vi "Configuration.Writer.Test.vi"() -> ()   [LabVIEW 2017, in "Measurement.Free.lvclass"]
uses:
  Measurement.Free.lvclass
  Typedefs/Configuration--Cluster.ctl
  Typedefs/Configuration.Hardware--Cluster.ctl
  Typedefs/Configuration.SMU--Cluster.ctl
  SMU/Typedefs/Configuration--Cluster.ctl
  Typedefs/Configuration.LIA--Cluster.ctl
  LIA/Typedefs/Configuration--Cluster.ctl
  Typedefs/Configuration.OPM--Cluster.ctl
  OPM/Typedefs/Configuration--Cluster.ctl
  Typedefs/Configuration.OPA--Cluster.ctl
  OPA/Typedefs/Configuration--Cluster.ctl
  <vilib>/Utility/config.llb/NI_LVConfig.lvlib
  SMU/SMU.lvclass
  LIA/LIA.lvclass
  OPM/OPM.lvclass
  OPA/OPA.lvclass
panel:
  out "error out":errorcluster
  in  "Configuration":T1={"Measurement.Type"=enum."Free", "Configuration.Hardware"={"Configuration.SMU"={"SMU Model"="Keithley2600", "Configuration"={"VISA Resource"="GPIB0::26::INSTR", "Channel"="A"}}, "Configuration.LIA"={"LIA Model"="SR810", "Configuration"={"VISA Resource"="GPIB0::8::INSTR"}}, "Configuration.OPM"={"OPM Model"="ThorlabsPM400", "Configuration"={"VISA Resource"="USB0::0x1313::0x8075::P5001221::INSTR"}}, "Configuration.OPA"={"OPA Model"="OrpheusHP", "Configuration"={"Serial Number"="Orpheus-HP-Demo-8047"}}}}
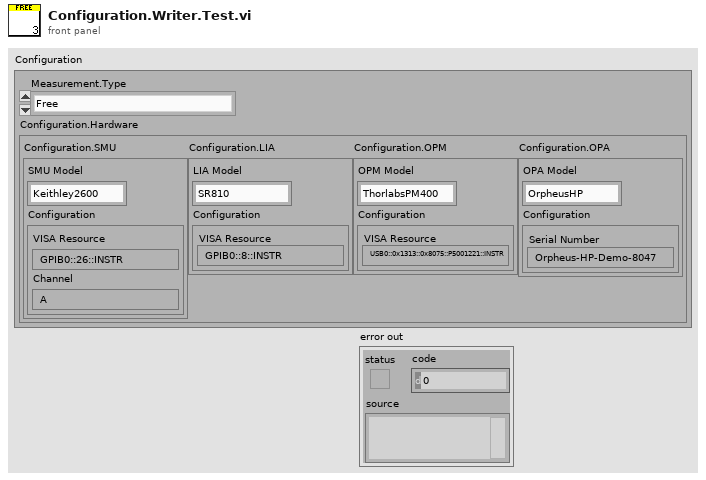
[diagram p1: front panel]
types:
  T1 = typedef "Measurement.Free.lvclass/Configuration--Cluster.ctl" = cluster{"Measurement.Type":enum16{"Free", "I/V Curve", "Wavelength sweeping", "Photocurrent mapping"}, "Configuration.Hardware":T2}
  T2 = typedef "Measurement.Free.lvclass/Configuration.Hardware--Cluster.ctl" = cluster{"Configuration.SMU":T3, "Configuration.LIA":T5, "Configuration.OPM":T7, "Configuration.OPA":T9}
  T3 = typedef "Measurement.Free.lvclass/Configuration.SMU--Cluster.ctl" = cluster{"SMU Model":string, "Configuration":T4}
  T4 = typedef "SMU.lvclass/Configuration--Cluster.ctl" = cluster{"VISA Resource":string, "Channel":string}
  T5 = typedef "Measurement.Free.lvclass/Configuration.LIA--Cluster.ctl" = cluster{"LIA Model":string, "Configuration":T6}
  T6 = typedef "LIA.lvclass/Configuration--Cluster.ctl" = cluster{"VISA Resource":string}
  T7 = typedef "Measurement.Free.lvclass/Configuration.OPM--Cluster.ctl" = cluster{"OPM Model":string, "Configuration":T8}
  T8 = typedef "OPM.lvclass/Configuration--Cluster.ctl" = cluster{"VISA Resource":string}
  T9 = typedef "Measurement.Free.lvclass/Configuration.OPA--Cluster.ctl" = cluster{"OPA Model":string, "Configuration":T10}
  T10 = typedef "OPA.lvclass/Configuration--Cluster.ctl" = cluster{"Serial Number":string}
  T11 = typedef "NI_LVConfig.lvlib/Config Data RefNum.ctl" = refnum<k1>
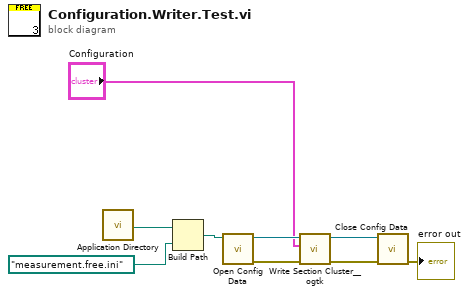
[diagram p0: block diagram]
diagram:
  n1 = call <vilib>:"Application Directory.vi"() -> ("Application Directory"=w9:path)
  n2 = Build Path(base path=w9, name or relative path=path "measurement.free.ini") -> (appended path=w7:path)
  n3 = call <vilib>:"Open Config Data.vi"("configuration file path"=w7) -> ("error out"=w6:errorcluster, "refnum"=w3:T11)  [unwired: 8 in, 1 out]
  n4 = call <userlib>:"Write Section Cluster__ogtk.vi"("error in (no error)"=w6, "Section Formatted Cluster"="Configuration", "refnum"=w3) -> ("error out"=w5:errorcluster, "dup refnum"=w4:T11)  [unwired: 7 in]
  n5 = call <vilib>:"Close Config Data.vi"("error in (no error)"=w5, "refnum"=w4) -> ("error out"=→"error out":errorcluster)  [unwired: 8 in, 1 out]
